vi "C Series Module EEPROM Information.vi"(8 "error in":errorcluster, 10 "Module":u16, 11 "Refnum in":refnum<k20>) -> (0 "error out":errorcluster, 2 "Module Information":T1 {"Module Code" format="%.0x"}, 3 "Refnum out":refnum<k20>)   [LabVIEW 2015, in "SMI.lvlib" / "C Series Module.lvclass"]
uses:
  C Series Module.lvclass
  Module/Controls/ModuleInformation.ctl
  <vilib>/Utility/error.llb/Error Cluster From Error Code.vi
  <vilib>/rvi/errors/niLvFpgaAdjustHostInterfaceError.vi
  <vilib>/rvi/interface/nirviReadWriteControl/nirviReadWriteControl.xnode
  <vilib>/ErrorRing/Error Ring.xnode
  NiFpgaLv.dll
  <vilib>/rvi/interface/Simulation/niFpgaSimulationCallBeginRW.vi
  Module/Module.lvclass
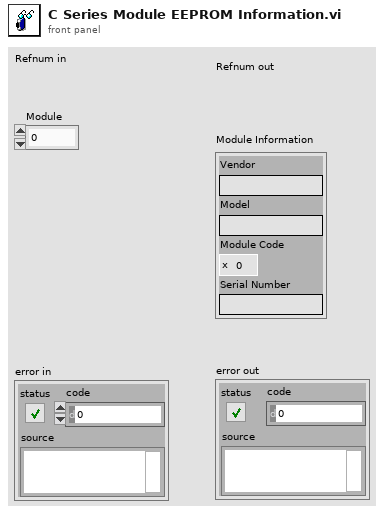
[diagram p1: front panel]
types:
  T1 = typedef "SMI.lvlib/Module.lvclass/ModuleInformation.ctl" = cluster{"Vendor":string, "Model":string, "Module Code":u16, "Serial Number":string}
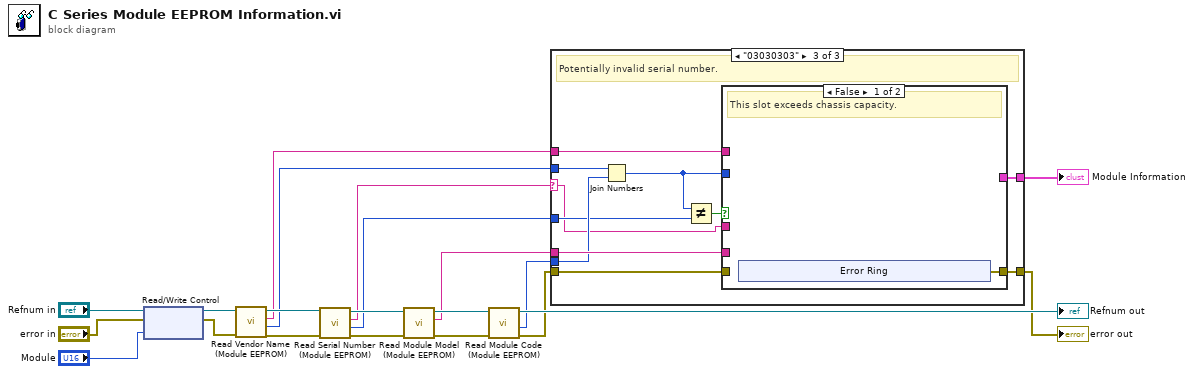
[diagram p0: block diagram]
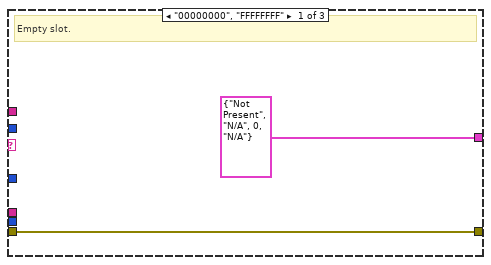
[diagram p2: hidden frame]
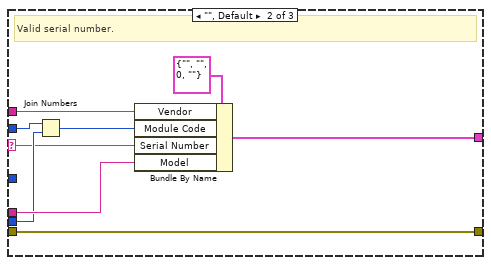
[diagram p3: hidden frame]
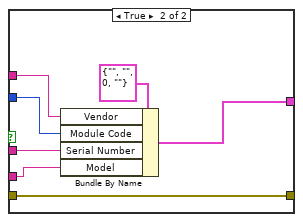
[diagram p4: hidden frame]
diagram:
  n1 = xnode "Read/Write Control"("FPGA VI Reference In"="Refnum in", "error in"="error in", "Module"="Module") -> ("FPGA VI Reference Out"=w15:refnum<k20>, "error out"=w16:errorcluster)
  n2 = call "Read Vendor Name (Module EEPROM).vi"("error in"=w16, "Refnum in"=w15) -> ("error out"=w18:errorcluster, "Vendor ID"=w8:u16, "Vendor Name"=w5:string, "Refnum out"=w19:refnum<k20>)  [unwired: 6 in]
  n3 = call "Read Serial Number (Module EEPROM).vi"("error in"=w18, "Refnum in"=w19) -> ("error out"=w21:errorcluster, "Serial Number"=w6:u32, "Serial Number String"=w12:string, "Refnum out"=w20:refnum<k20>)  [unwired: 6 in]
  n4 = call "Read Module Model (Module EEPROM).vi"("error in"=w21, "Refnum in"=w20) -> ("error out"=w11:errorcluster, "Module Model"=w4:string, "Refnum out"=w10:refnum<k20>)  [unwired: 7 in]
  n5 = call "Read Module Code (Module EEPROM).vi"("error in"=w11, "Refnum in"=w10) -> ("error out"=w3:errorcluster, "Module ID"=w7:u16, "Refnum out"=→"Refnum out":refnum<k20>)  [unwired: 6 in, 1 out]
  n6 = case shown="\"03030303\"" w12 {
    selector: w12 -> [_ w24 w34]
    tunnel: w5 -> [_ w32 w43]
    tunnel: w4 -> [_ w31 w42]
    tunnel: [T1 {"Vendor"="Not Present", "Model"="N/A", "Module Code"=0, "Serial Number"="N/A"} ("cRIO Module Information") w30 w33] -> w1
    tunnel: w7 -> [_ w29 w41]
    tunnel: w8 -> [_ w28 w40]
    tunnel: w6 -> [_ _ w35]
    tunnel: w3 -> [w23 w25 w38]
    tunnel: [w23 w25 w37] -> w2
    frame "00000000", "FFFFFFFF" {
      # "Empty slot."
    }
    frame "", Default {
      # "Valid serial number."
      n7 = Join Numbers(hi=w28, lo=w29) -> ((hi.lo)=w26:u32)
      n8 = Bundle By Name(cluster=T1 {"Vendor"="", "Model"="", "Module Code"=0, "Serial Number"=""} ("Module Information"), "Vendor"=w32, "Module Code"=w26, "Serial Number"=w24, "Model"=w31) -> (w30:T1)
    }
    frame "03030303" {
      # "Potentially invalid serial number."
      n9 = Join Numbers(hi=w40, lo=w41) -> ((hi.lo)=w36:u32)
      n10 = Not Equal?(x=w36, y=w35) -> (x != y?=w39:bool)
      n11 = case shown="False" w39 {
        tunnel: w43 -> [_ w55]
        tunnel: w42 -> [_ w54]
        tunnel: [_ w53] -> w33
        tunnel: w34 -> [_ w52]
        tunnel: w36 -> [_ w50]
        tunnel: w38 -> [_ w49]
        tunnel: [w44 w49] -> w37
        frame False {
          # "This slot exceeds chassis capacity."
          n12 = xnode "Error Ring"() -> ("error out"=w44:errorcluster)
        }
        frame True {
          n13 = Bundle By Name(cluster=T1 {"Vendor"="", "Model"="", "Module Code"=0, "Serial Number"=""} ("Module Information"), "Vendor"=w55, "Module Code"=w50, "Serial Number"=w52, "Model"=w54) -> (w53:T1)
        }
      }
    }
  }
  "error out" <- w2
  "Module Information" <- w1
